vi "Destroy.vi"(8 "error in (no error)":errorcluster, 11 "Object in":refnum<class "Object.lvclass">) -> (0 "error out":errorcluster)   [LabVIEW 2019, in "HierDAL Library.lvlib" / "Models.lvlib" / "Object.lvclass"]
uses:
  Object.lvclass
  Object.lvclass/Object.ctl
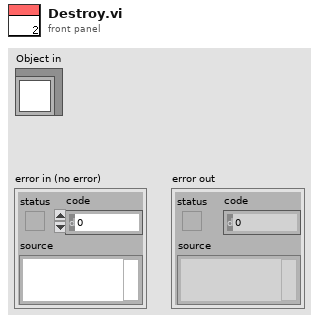
[diagram p1: front panel]
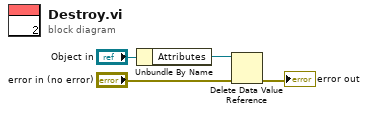
[diagram p0: block diagram]
diagram:
  n1 = Unbundle By Name("Object in") -> ("Attributes"=w3:refnum<data-value>)
  n2 = Delete Data Value Reference(data value reference=w3, error in="error in (no error)") -> (error out=→"error out":errorcluster)  [unwired: 1 out]
